vi "Bloomy BS120x Discovery Example.vi"(8 "error in (no error)":errorcluster, 11 "Allow Selection":bool) -> (0 "error out":errorcluster, 1 "Canceled":bool, 2 "Selected Device":T1, 3 "Discovered Devices":T1[](array[typedef]))   [LabVIEW 2021]
uses:
  src/Public/New BS120x Device/DiscoveredDevice.ctl
  src/TypeDefs/UnitType.ctl
  src/TypeDefs/Protocol.ctl
  src/BS120x Driver.lvlib
  src/BS120x.lvclass
panel:
  in  "Select":bool
  in  "stop":bool
  in  "Bloomy Cell Simulators":i32(listbox)=-1
  in  "Discover":bool
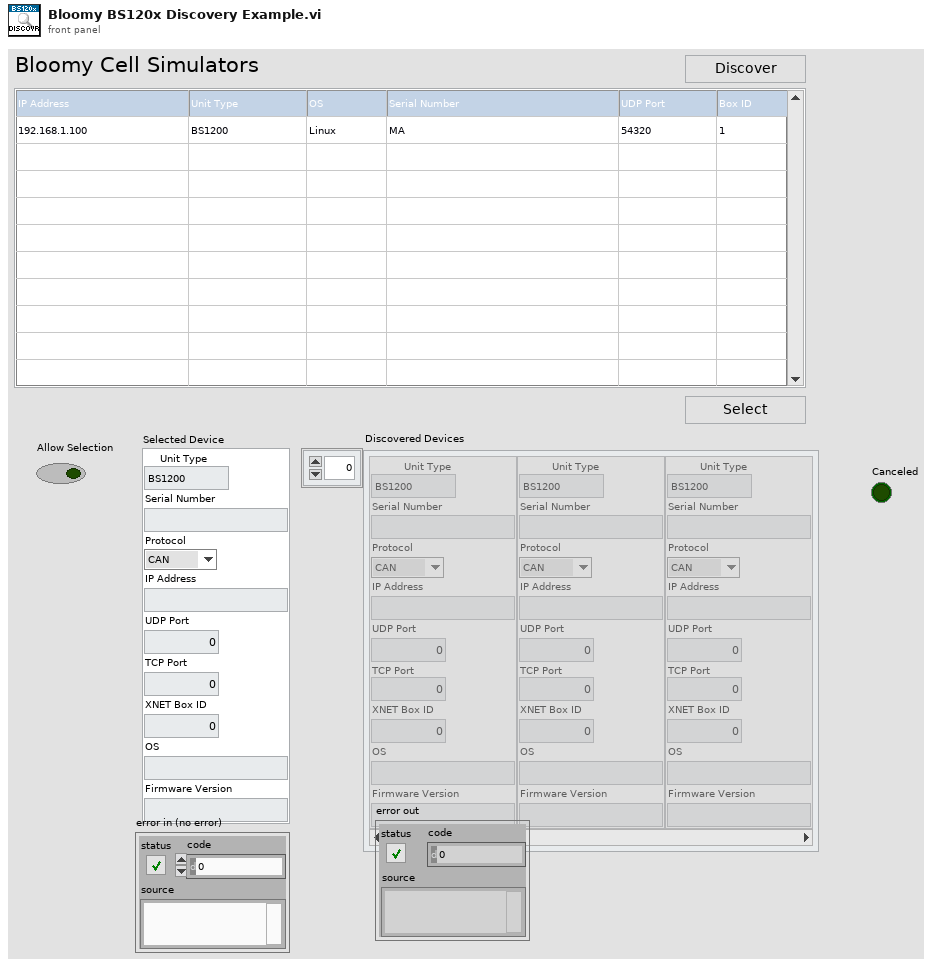
[diagram p1: front panel]
types:
  T1 = typedef "BS120x Driver.lvlib/DiscoveredDevice.ctl" = cluster{"Unit Type":T2, "Serial Number":string, "Protocol":T3, "IP Address":string, "UDP Port":u16, "TCP Port":u16, "XNET Box ID":u8, "OS":string, "Firmware Version":string}
  T2 = typedef "BS120x Driver.lvlib/BS120x.lvclass/UnitType.ctl" = enum16{"BS1200", "BS1201"}
  T3 = typedef "BS120x Driver.lvlib/BS120x.lvclass/Protocol.ctl" = enum16{"CAN", "Ethernet"}
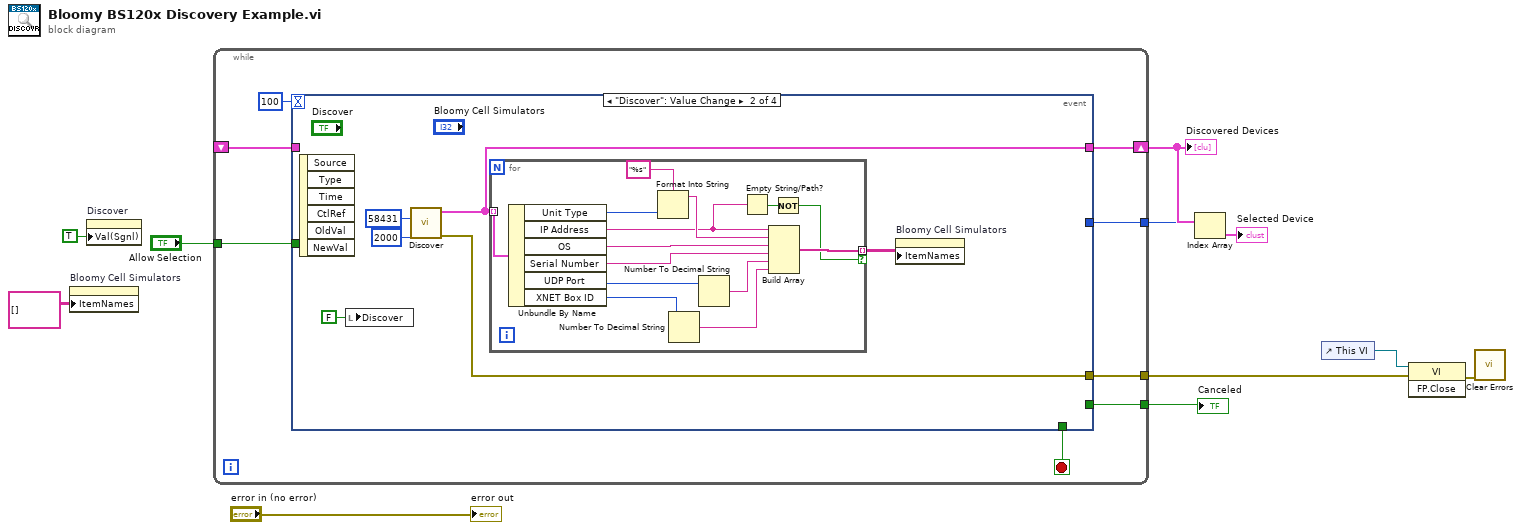
[diagram p0: block diagram]
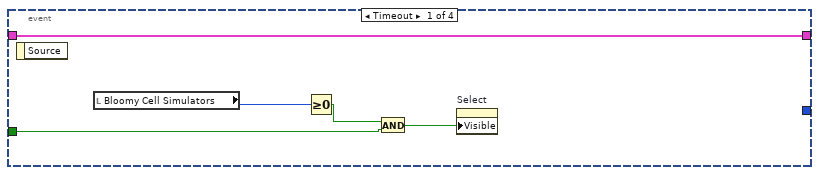
[diagram p2: hidden frame]
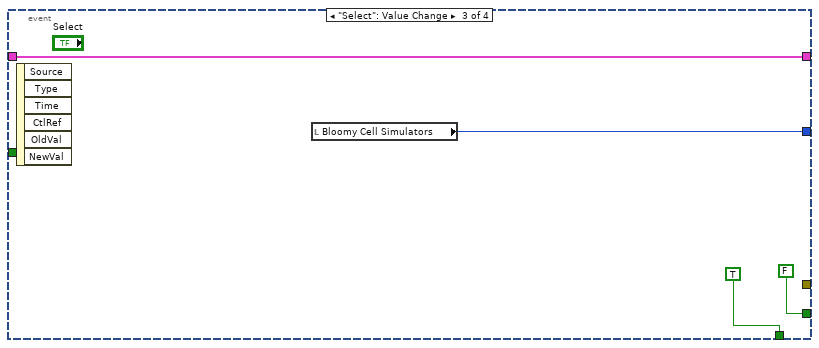
[diagram p3: hidden frame]
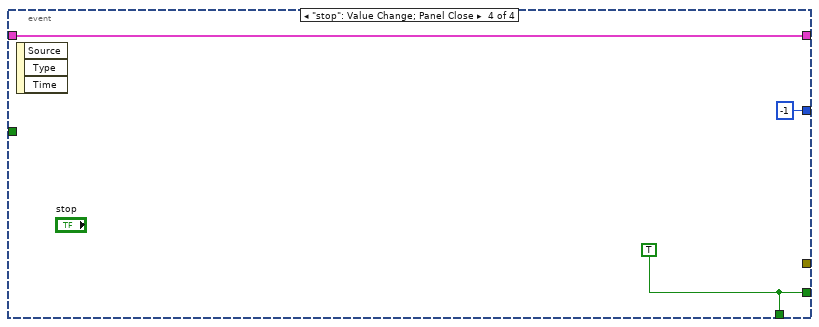
[diagram p4: hidden frame]
diagram:
  n1 = property on="Bloomy Cell Simulators" class="MCListbox (strict)"("ItemNames"=string[][] [] ("Item Names")) -> ()  [unwired: 2 in, 2 out]
  n2 = property on="Discover" class="Bool (strict)"("Val(Sgnl)"=TRUE ("Value (Signaling)")) -> ()  [unwired: 2 in, 2 out]
  n3 = while {
    shift-right: [w18] -> w9
    shift-left: _ -> [w17]
    tunnel: [w16] -> w8
    tunnel: [w15] -> w6
    tunnel: [w14] -> w4
    tunnel: "Allow Selection" -> [w12]
    stop <- w19 stop-if-true
    n4 = event shown="[1] \"Discover\": Value Change" {
      selector: _ -> [_ _ _ _]
      dyn-events: _ -> [_ _ _ _]
      timeout: 100 -> [_ _ _ _]
      tunnel: [_ _ TRUE w49] -> w19
      tunnel: [w24 w26 w48 w51] -> w18
      tunnel: w17 -> [w24 _ w48 w51]
      tunnel: [_ _ w47 -1 ("Bloomy Cell Simulators")] -> w16
      tunnel: [_ _ FALSE w49] -> w15
      tunnel: [_ w25 _ _] -> w14
      tunnel: w12 -> [w21 _ _ _]
      event Timeout {
        n5 = event-data() -> ()  [unwired: 1 in, 1 out]
        n6 = local read "Bloomy Cell Simulators"() -> (w23:i32)
        n7 = Greater Or Equal To 0?(x=w23) -> (x >= 0?=w22:bool)
        n8 = And(x=w22, y=w21) -> (x .and. y?=w20:bool)
        n9 = property on="Select" class="Bool (strict)"("Visible"=w20) -> ()  [unwired: 2 in, 2 out]
      }
      event "Discover": Value Change {
        n10 = event-data() -> ()  [unwired: 1 in, 6 out]
        n11 = local write "Discover"(FALSE ("Discover")) -> ()
        n12 = call "Discover.vi"("Timeout (ms)"=2000, "Port"=58431) -> ("error out"=w25:errorcluster, "Discovered Devices"=w26:T1[])  [unwired: 8 in]
        n13 = for {
          tunnel: w26 -> [w44] mode=indexing
          tunnel: [w38] -> w29 mode=indexing if=w32
          n14 = Unbundle By Name(w44) -> ("Unit Type"=w42:T2, "IP Address"=w33:string, "OS"=w31:string, "Serial Number"=w36:string, "UDP Port"=w37:u16, "XNET Box ID"=w40:u8)
          n15 = Format Into String(format string="%s", w42) -> (resulting string=w35:string)  [unwired: 2 in, 1 out]
          n16 = Number To Decimal String(number=w40) -> (decimal integer string=w39:string)  [unwired: 1 in]
          n17 = Number To Decimal String(number=w37) -> (decimal integer string=w41:string)  [unwired: 1 in]
          n18 = Empty String/Path?(string/path=w33) -> (empty?=w34:bool)
          n19 = Build Array(w33, w35, w31, w36, w41, w39) -> (w38:string[])
          n20 = Not(x=w34) -> (.not. x?=w32:bool)
        }
        n21 = property on="Bloomy Cell Simulators" class="MCListbox (strict)"("ItemNames"=w29) -> ()  [unwired: 2 in, 2 out]
      }
      event "Select": Value Change {
        n22 = event-data() -> ()  [unwired: 1 in, 6 out]
        n23 = local read "Bloomy Cell Simulators"() -> (w47:i32)
      }
      event "stop": Value Change; Panel Close {
        w49 = TRUE
        n24 = event-data() -> ()  [unwired: 1 in, 3 out]
      }
    }
  }
  "Discovered Devices" <- w9
  "Canceled" <- w6
  n25 = Index Array(array=w9, index=w8) -> (element=→"Selected Device":T1)
  n26 = control-ref of="This VI"() -> (w5:refnum<vi>)
  n27 = invoke class="VI" method="FP.Close"(reference=w5, error in=w4) -> (error out=w3:errorcluster)  [unwired: 1 in, 2 out]
  n28 = call <vilib>:"Clear Errors.vi"("error in (no error)"=w3) -> ()  [unwired: 5 in, 2 out]
  "error out" <- "error in (no error)"
